vi "LIN Write.vi"(3 "Error IN":errorcluster, 4 "Tx Msg":u8[][](array[numeric]) format="%.0x", 5 "LIN Device IN":T1={"Master Frame(3C)"="MasterReq\nSPA3414_ConfigurationsCMAGeely_CEMCALYPSOSDB34XX0Cfg_LIN3_190709_", "Slave Frame(3D)"="SlaveResp\nSPA3414_ConfigurationsCMAGeely_CEMCALYPSOSDB34XX0Cfg_LIN3_190709_", "Request Schedule"="CEMLIN3DiagRequestSchedule\nSPA3414_ConfigurationsCMAGeely_CEMCALYPSOSDB34XX0Cfg_LIN3_190709_", "Response Schedule"="CEMLIN3DiagResponseSchedule\nSPA3414_ConfigurationsCMAGeely_CEMCALYPSOSDB34XX0Cfg_LIN3_190709_", "Frame Write SCU"="", "Frame Read SCU"="", "LIN Name"=""}, 6 "NAD":u8) -> (0 "error out":errorcluster, 1 "Array":u8[](array[numeric]), 2 "LIN Device OUT":T1={"Master Frame(3C)"="MasterReq\nSPA3414_ConfigurationsCMAGeely_CEMCALYPSOSDB34XX0Cfg_LIN3_190709_", "Slave Frame(3D)"="SlaveResp\nSPA3414_ConfigurationsCMAGeely_CEMCALYPSOSDB34XX0Cfg_LIN3_190709_", "Request Schedule"="CEMLIN3DiagRequestSchedule\nSPA3414_ConfigurationsCMAGeely_CEMCALYPSOSDB34XX0Cfg_LIN3_190709_", "Response Schedule"="CEMLIN3DiagResponseSchedule\nSPA3414_ConfigurationsCMAGeely_CEMCALYPSOSDB34XX0Cfg_LIN3_190709_", "Frame Write SCU"="", "Frame Read SCU"="", "LIN Name"=""})   [LabVIEW 2018]
uses:
  LIN Device.ctl
  <vilib>/xnet/xnet.llb/XNET Frame LIN.ctl
  <vilib>/xnet/xnet.llb/XNET Frame Type LIN.ctl
  <vilib>/xnet/xnet.llb/XNET Write (State LIN Schedule Change).vi
  <vilib>/xnet/xnet.llb/XNET Write (Frame LIN).vi
  <vilib>/xnet/xnet.llb/XNET Wait (Transmit Complete).vi
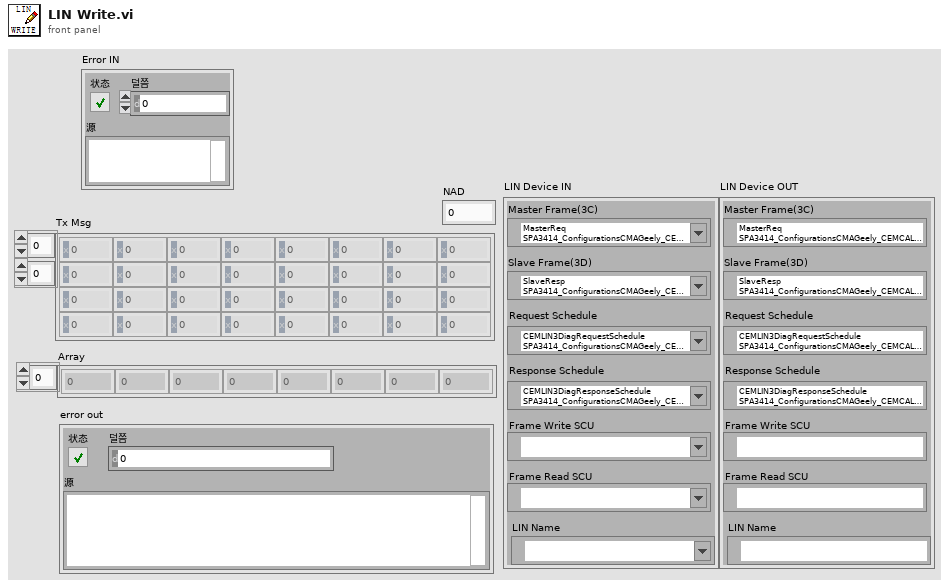
[diagram p1: front panel]
types:
  T1 = typedef "LIN Device.ctl" = cluster{"Master Frame(3C)":refnum<k21>, "Slave Frame(3D)":refnum<k21>, "Request Schedule":refnum<k21>, "Response Schedule":refnum<k21>, "Frame Write SCU":refnum<k21>, "Frame Read SCU":refnum<k21>, "LIN Name":refnum<k21>}
  T2 = typedef "XNET Frame LIN.ctl" = cluster{"timestamp":timestamp, "payload":u8[], "identifier":u32, "type":T3, "event ID":u8, "event slot?":bool, "echo?":bool}
  T3 = typedef "XNET Frame Type LIN.ctl" = u8
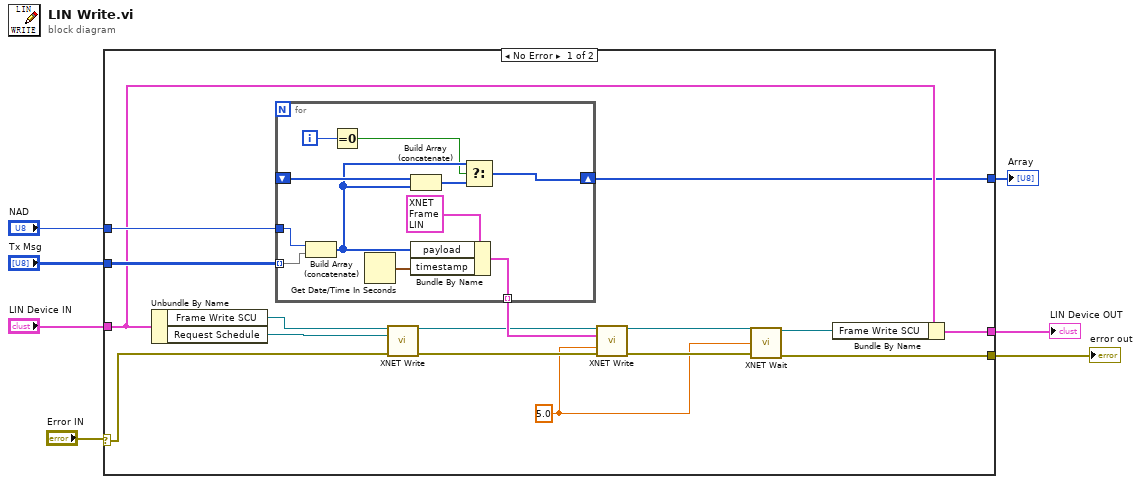
[diagram p0: block diagram]
diagram:
  n1 = case shown="No Error" "Error IN" {
    selector: "Error IN" -> [w21 w35]
    tunnel: "LIN Device IN" -> [w12 w36]
    tunnel: "Tx Msg" -> [w20 _]
    tunnel: "NAD" -> [w19 _]
    tunnel: [w10 _] -> w3
    tunnel: [w9 w36] -> w2
    tunnel: [w8 w35] -> w1
    frame No Error {
      w13 = 5.0 ("timeout (10)")
      n2 = Unbundle By Name(w12) -> ("Frame Write SCU"=w22:refnum<k21>, "Request Schedule"=w23:refnum<k21>)
      n3 = for {
        tunnel: w20 -> [w33] mode=indexing
        tunnel: w19 -> [w34]
        shift-right: [w30] -> w10
        shift-left: _ -> [w31]
        tunnel: [w25] -> w18 mode=indexing
        i -> [w27]
        n4 = Build Array (concatenate)(w34, w33) -> (w29:u8[])
        n5 = Equal To 0?(x=w27) -> (x = 0?=w26:bool)
        n6 = Get Date/Time In Seconds() -> (seconds since 1Jan1904=w32:timestamp)
        n7 = Build Array (concatenate)(w31, w29) -> (w28:u8[])
        n8 = Bundle By Name(cluster=T2 {"timestamp"=timestamp(0 s since 1904-01-01), "payload"=[], "identifier"=0, "type"=64, "event ID"=0, "event slot?"=FALSE, "echo?"=FALSE} ("LIN frame"), "payload"=w29, "timestamp"=w32) -> (w25:T2)
        n9 = Select(t=w29, s=w26, f=w28) -> (s? t:f=w30:u8[])
      }
      n10 = call-poly <vilib>:"XNET Write.vi"("session in"=w22, "data"=w23, "error in (no error)"=w21) -> ("session out"=w17:refnum<k21>, "error out"=w16:errorcluster)  [unwired: 11 in]
      n11 = call-poly <vilib>:"XNET Write.vi"("session in"=w17, "data"=w18, "timeout (10)"=w13, "error in (no error)"=w16) -> ("session out"=w15:refnum<k21>, "error out"=w14:errorcluster)  [unwired: 10 in]
      n12 = call-poly <vilib>:"XNET Wait.vi"("session in"=w15, "timeout (10)"=w13, "error in (no error)"=w14) -> ("session out"=w11:refnum<k21>, "error out"=w8:errorcluster)  [unwired: 11 in]
      n13 = Bundle By Name(cluster=w12, "Frame Write SCU"=w11) -> (w9:T1)
    }
    frame Error {
    }
  }
  "Array" <- w3
  "LIN Device OUT" <- w2
  "error out" <- w1
